vi "JoelReflectivityModel.vi"(8 "error in (no error)":errorcluster, 10 "Parameters":dbl[](array[numeric]), 11 "x":dbl format="%#_13g") -> (0 "error out":errorcluster, 3 "y":dbl format="%#_13g")   [LabVIEW 2016]
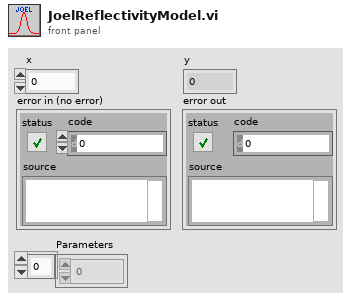
[diagram p1: front panel]
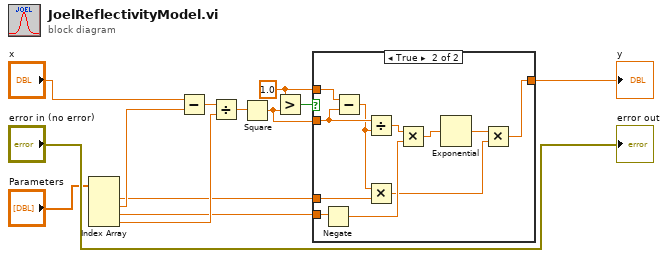
[diagram p0: block diagram]
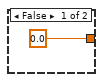
[diagram p2: hidden frame]
diagram:
  w5 = 1.0 ("x")
  n1 = Index Array(array="Parameters") -> (element #1=w7:dbl, element #2=w12:dbl, element #3=w6:dbl, element #4=w10:dbl)  [unwired: 4 in]
  n2 = Subtract(x="x", y=w12) -> (x-y=w11:dbl)
  n3 = Divide(x=w11, y=w10) -> (x/y=w9:dbl)
  n4 = Square(x=w9) -> (x^2=w4:dbl)
  n5 = Greater?(x=w5, y=w4) -> (0:w8:bool)
  n6 = case shown="True" w8 {
    tunnel: [0.0 ("y") w15] -> w3
    tunnel: w7 -> [_ w19]
    tunnel: w6 -> [_ w23]
    tunnel: w5 -> [_ w25]
    tunnel: w4 -> [_ w24]
    frame False {
    }
    frame True {
      n7 = Negate(x=w23) -> (-x=w21:dbl)
      n8 = Subtract(x=w25, y=w24) -> (x-y=w18:dbl)
      n9 = Divide(x=w24, y=w18) -> (x/y=w22:dbl)
      n10 = Multiply(x=w18, y=w19) -> (x*y=w16:dbl)
      n11 = Multiply(x=w22, y=w21) -> (x*y=w20:dbl)
      n12 = Exponential(1:w20) -> (0:w17:dbl)
      n13 = Multiply(x=w17, y=w16) -> (x*y=w15:dbl)
    }
  }
  "y" <- w3
  "error out" <- "error in (no error)"
